vi "OK sur derivee.vi"() -> ()   [LabVIEW 2020, in "Library Commun.lvlib" / "Nodon_ZCR.lvclass"]
uses:
  Nodon_ZCR.lvclass
  Nodon_ZCR.lvclass/Nodon_ZCR.ctl
panel:
  in  "data 4":waveform(dbl)[](graph)=[{"t0"=timestamp(3707890383.8976955 s since 1904-01-01), "dt"=9.999999999999999e-05, "Y"=array[20000 elements], "attributes"=variant("NI_ChannelName"=variant(string "Tension_0"), "NI_UnitDescription"=variant(string "Volts"))}, {"t0"=timestamp(3707890383.8977456 s since 1904-01-01), "dt"=9.999999999999999e-05, "Y"=array[20000 elements], "attributes"=variant("NI_ChannelName"=variant(string "Tension_1"), "NI_UnitDescription"=variant(string "Volts"))}] caption="calibrer"
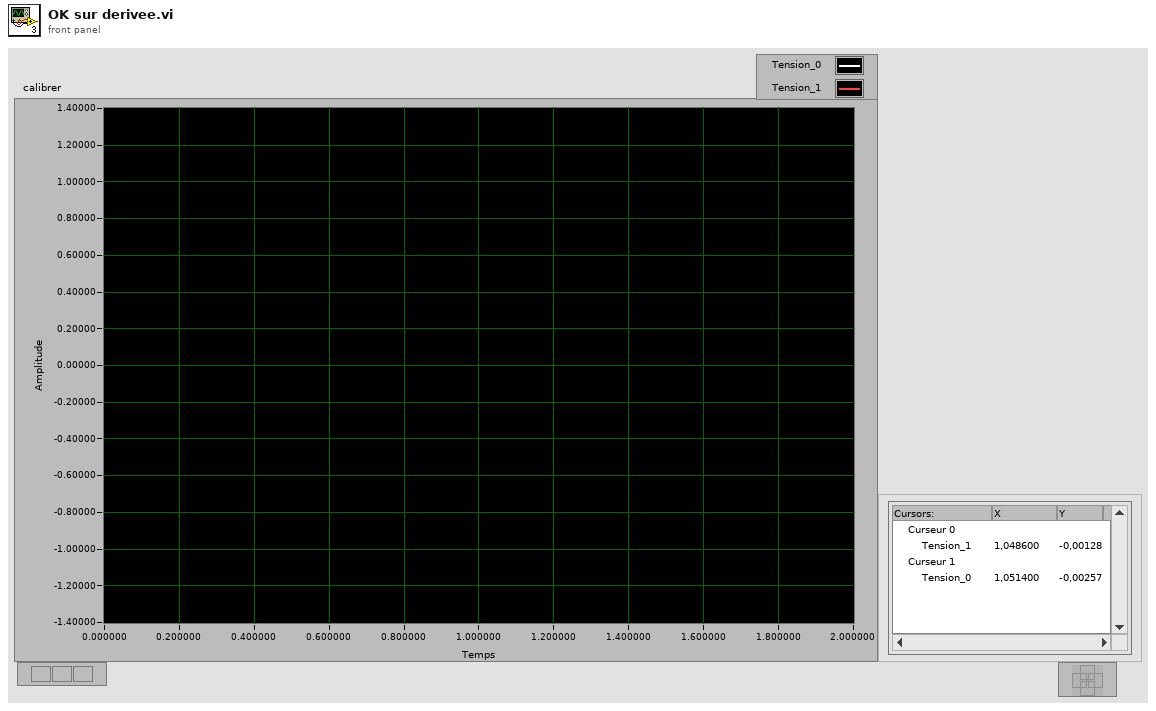
[diagram p1: front panel]
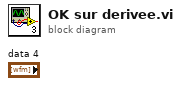
[diagram p0: block diagram]
diagram:
